vi "Check Status (No Objects).vi"(8 "error in (no error)":errorcluster, 11 "Cluster In":T1 {"Frequency Mode" items=["CW", "Fixed", "Stepped Sweep", "List Sweep"]; "Amplitude Mode" items=["Fixed", "Stepped Sweep", "List Sweep"]}) -> (0 "error out":errorcluster, 1 "Status":string, 2 "Ready?":bool, 3 "Cluster Out":T1 {"Frequency Mode" items=["CW", "Fixed", "Stepped Sweep", "List Sweep"]; "Amplitude Mode" items=["Fixed", "Stepped Sweep", "List Sweep"]})   [LabVIEW 2009]
doc: "(Dynamic) Check if the instrument is powered on and update its member data with the instrument's current status. Optionally return a text status message."
uses:
  Global/GPIB Numbers.vi
  Agilent PSG MXG Series/Agilent PSG MXG Series.lvlib
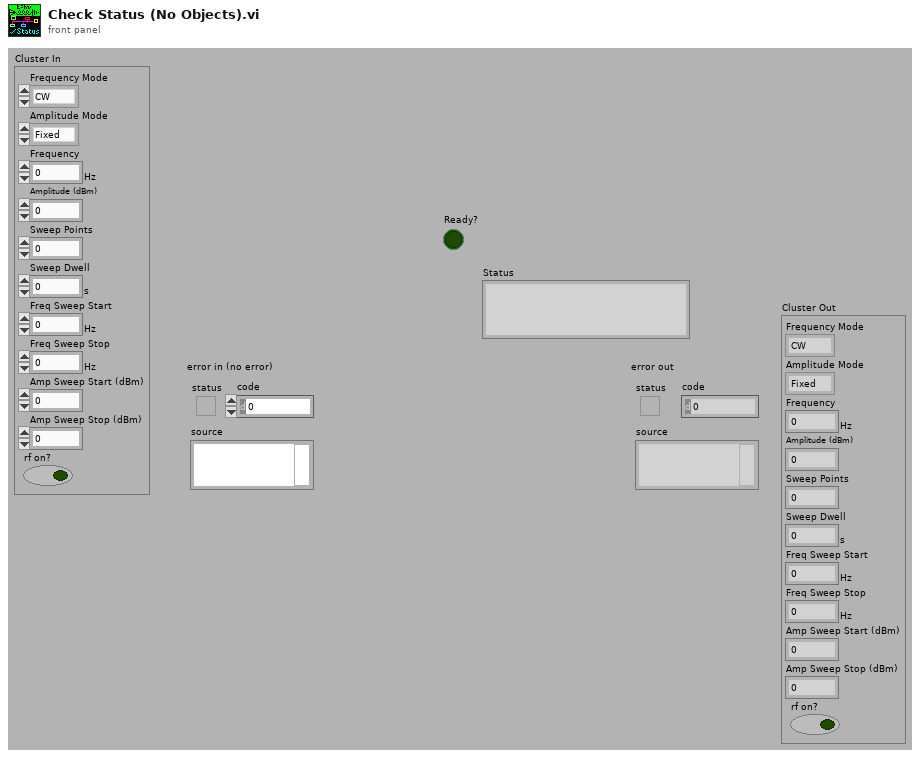
[diagram p1: front panel]
types:
  T1 = cluster{"Frequency Mode":u16, "Amplitude Mode":u16, "Frequency":dbl[unit], "Amplitude (dBm)":dbl, "Sweep Points":i32, "Sweep Dwell":dbl[unit], "Freq Sweep Start":dbl[unit], "Freq Sweep Stop":dbl[unit], "Amp Sweep Start (dBm)":dbl, "Amp Sweep Stop (dBm)":dbl, "rf on?":bool}
  T2 = typedef "GPIB Type Def.ctl" = cluster{"Name":string, "bus":dbl, "GPIB":dbl, "GPIB as string":string, "byte":i32, "VISA Resource Name":refnum<visa-resource-name>}
  T3 = enum16{"CW", "Fixed", "Stepped Sweep", "List Sweep"}
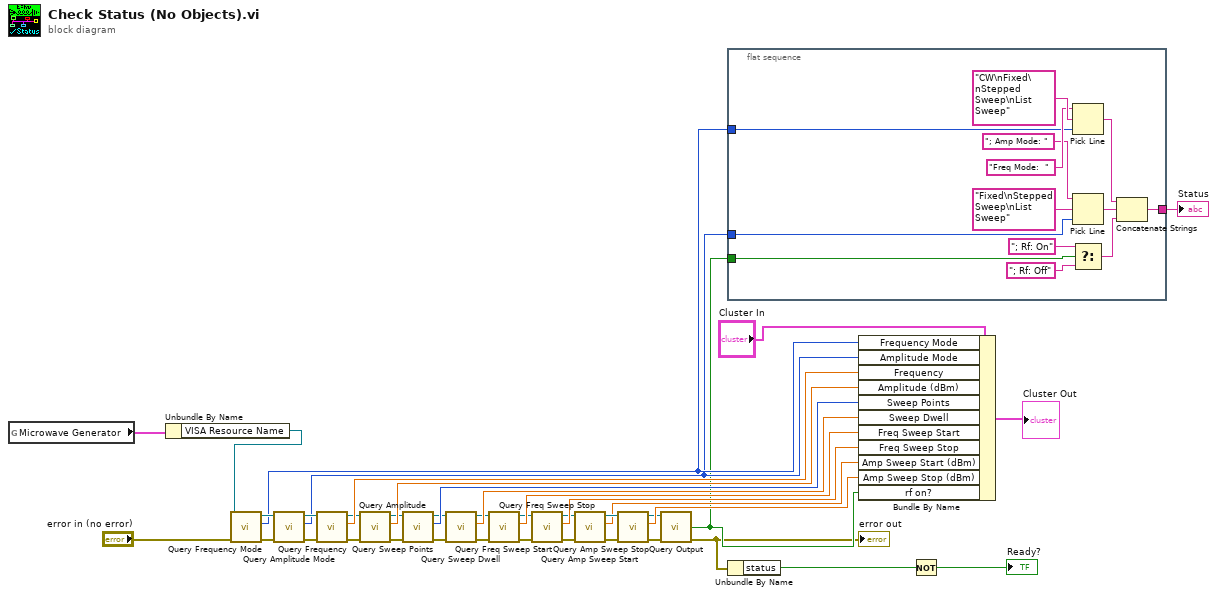
[diagram p0: block diagram]
diagram:
  n1 = global read "GPIB Numbers.vi" "Microwave Generator"() -> (w5:T2)
  n2 = Unbundle By Name(w5) -> ("VISA Resource Name"=w4:refnum<visa-resource-name>)
  n3 = call "Query Frequency Mode.vi"("error in (no error)"="error in (no error)", "VISA resource name"=w4) -> ("error out"=w8:errorcluster, "Frequency Mode"=w11:T3, "VISA resource name out"=w39:refnum<visa-resource-name>)  [unwired: 7 out]
  n4 = call "Query Amplitude Mode.vi"("error in (no error)"=w8, "VISA resource name"=w39) -> ("error out"=w37:errorcluster, "Amplitude Mode"=w10:enum16{"Fixed", "Stepped Sweep", "List Sweep"}, "VISA resource name out"=w38:refnum<visa-resource-name>)  [unwired: 7 out]
  n5 = call "Query Frequency.vi"("error in (no error)"=w37, "VISA resource name"=w38) -> ("error out"=w34:errorcluster, "Frequency"=w36:dbl[unit], "VISA resource name out"=w35:refnum<visa-resource-name>)  [unwired: 7 out]
  n6 = call "Query Amplitude.vi"("error in (no error)"=w34, "VISA resource name"=w35) -> ("error out"=w31:errorcluster, "Amplitude (dBm)"=w33:dbl, "VISA resource name out"=w32:refnum<visa-resource-name>)  [unwired: 7 out]
  n7 = call "Query Sweep Points.vi"("error in (no error)"=w31, "VISA resource name"=w32) -> ("error out"=w28:errorcluster, "Number of Sweep Points"=w30:i32, "VISA resource name out"=w29:refnum<visa-resource-name>)  [unwired: 7 out]
  n8 = call "Query Sweep Dwell.vi"("error in (no error)"=w28, "VISA resource name"=w29) -> ("error out"=w25:errorcluster, "Sweep Dwell Time"=w27:dbl[unit], "VISA resource name out"=w26:refnum<visa-resource-name>)  [unwired: 7 out]
  n9 = call "Query Freq Sweep Start.vi"("error in (no error)"=w25, "VISA resource name"=w26) -> ("error out"=w22:errorcluster, "Frequency Sweep Start"=w24:dbl[unit], "VISA resource name out"=w23:refnum<visa-resource-name>)  [unwired: 7 out]
  n10 = call "Query Freq Sweep Stop.vi"("error in (no error)"=w22, "VISA resource name"=w23) -> ("error out"=w17:errorcluster, "Frequency Sweep Stop"=w21:dbl[unit], "VISA resource name out"=w18:refnum<visa-resource-name>)  [unwired: 7 out]
  n11 = call "Query Amp Sweep Start.vi"("error in (no error)"=w17, "VISA resource name"=w18) -> ("error out"=w19:errorcluster, "Amplitude Sweep Start (dBm)"=w16:dbl, "VISA resource name out"=w20:refnum<visa-resource-name>)  [unwired: 7 out]
  n12 = call "Query Amp Sweep Stop.vi"("error in (no error)"=w19, "VISA resource name"=w20) -> ("error out"=w13:errorcluster, "Amplitude Sweep Stop (dBm)"=w15:dbl, "VISA resource name out"=w14:refnum<visa-resource-name>)  [unwired: 7 out]
  n13 = call "Query Output.vi"("error in (no error)"=w13, "VISA resource name"=w14) -> ("error out"=w2:errorcluster, "Output On?"=w9:bool)  [unwired: 8 out]
  "error out" <- w2
  n14 = flat-sequence {
    tunnel: [w51] -> w12
    tunnel: w11 -> [w47]
    tunnel: w10 -> [w46]
    tunnel: w9 -> [w42]
    frame #0 {
      n15 = Pick Line(string ("")="Freq Mode:  ", multi-line string="CW\nFixed\nStepped Sweep\nList Sweep", line index=w47) -> (output string=w52:string)
      n16 = Pick Line(string ("")="; Amp Mode: ", multi-line string="Fixed\nStepped Sweep\nList Sweep", line index=w46) -> (output string=w45:string)
      n17 = Select(t="; Rf: On" ("string (\"\")"), s=w42, f="; Rf: Off" ("string (\"\")")) -> (s? t:f=w41:string)
      n18 = Concatenate Strings(w52, w45, w41) -> (w51:string)
    }
  }
  n19 = Unbundle By Name(w2) -> ("status"=w40:bool)
  n20 = Bundle By Name(cluster="Cluster In", "Frequency Mode"=w11, "Amplitude Mode"=w10, "Frequency"=w36, "Amplitude (dBm)"=w33, "Sweep Points"=w30, "Sweep Dwell"=w27, "Freq Sweep Start"=w24, "Freq Sweep Stop"=w21, "Amp Sweep Start (dBm)"=w16, "Amp Sweep Stop (dBm)"=w15, "rf on?"=w9) -> (→"Cluster Out":T1)
  n21 = Not(x=w40) -> (.not. x?=→"Ready?":bool)
  "Status" <- w12
